vi "Load Layout.vi"(7 "SP_Main":refnum<vi>, 8 "error in (no error)":errorcluster, 11 "hse-config":refnum<class "config-base.lvclass">) -> (0 "error out":errorcluster, 3 "Layout out":T1)   [LabVIEW 2022 SP3, in "UI Manager.lvlib"]
doc: "Loads all the layout files and references and populates the subpanels as configured in UI Manager.ini\n\n____\nHAMPEL SOFTWARE ENGINEERING v2.6.0 (2023-12-19 10:54)"
uses:
  UI Manager.lvlib
  Layout References--cluster.ctl
  SubPanels--map.ctl
  SubPnl Map References--cluster.ctl
  Libraries/hse-libraries/Source/hse-configuration/config-base/config-base.lvclass
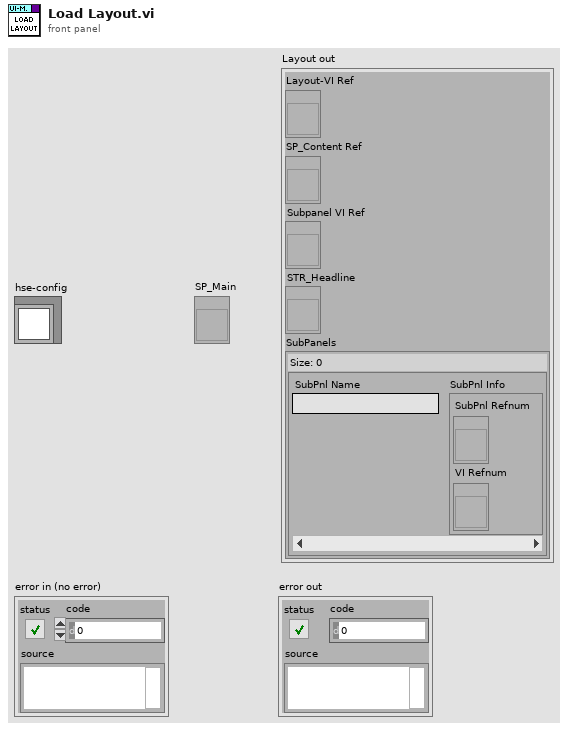
[diagram p1: front panel]
types:
  T1 = typedef "UI Manager.lvlib/Layout References--cluster.ctl" = cluster{"Layout-VI Ref":refnum<vi>, "SP_Content Ref":refnum<vi>, "Subpanel VI Ref":refnum<vi>, "STR_Headline":refnum<vi>, "SubPanels":T2}
  T2 = typedef "UI Manager.lvlib/SubPanels--map.ctl" = map{string, T3}
  T3 = typedef "UI Manager.lvlib/SubPnl Map References--cluster.ctl" = cluster{"SubPnl Refnum":refnum<vi>, "VI Refnum":refnum<vi>}
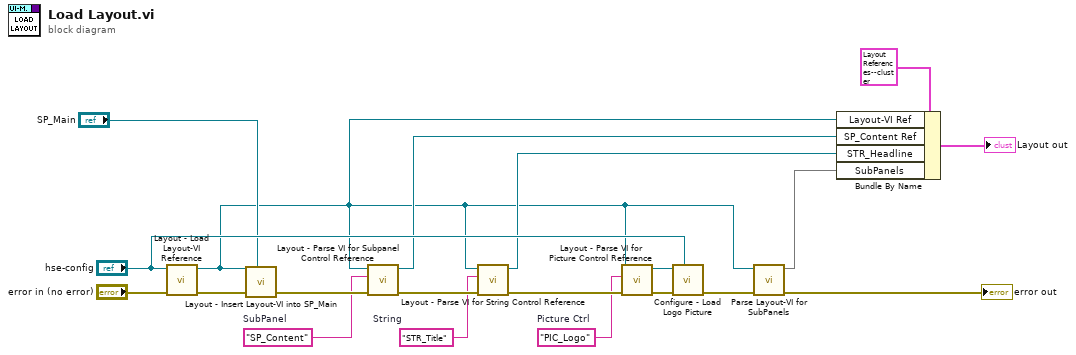
[diagram p0: block diagram]
diagram:
  w6 = "PIC_Logo"  # Picture Ctrl
  w9 = "STR_Title"  # String
  w16 = "SP_Content"  # SubPanel
  n1 = call "Layout - Load Layout-VI Reference.vi"("error in (no error)"="error in (no error)", "hse-config"="hse-config") -> ("error out"=w17:errorcluster, "Layout-VI Ref"=w2:refnum<vi>)  [unwired: 8 in]
  n2 = call "Layout - Insert Layout-VI into SP_Main.vi"("SubPanel in"="SP_Main", "error in (no error)"=w17, "Layout-VI Ref"=w2) -> ("error out"=w18:errorcluster)  [unwired: 8 in]
  n3 = call "Layout - Parse VI for Subpanel Control Reference.vi"("error in (no error)"=w18, "SubPanel Label"=w16, "VI in"=w2) -> ("error out"=w15:errorcluster, "SubPanel Ref"=w19:refnum<vi>)  [unwired: 7 in]
  n4 = call "Layout - Parse VI for String Control Reference.vi"("error in (no error)"=w15, "String Label"=w9, "VI in"=w2) -> ("error out"=w10:errorcluster, "String Reference"=w8:refnum<vi>)  [unwired: 7 in]
  n5 = call "Layout - Parse VI for Picture Control Reference.vi"("error in (no error)"=w10, "Picture Control Label"=w6, "VI in"=w2) -> ("error out"=w7:errorcluster, "Picture Control Ref"=w5:refnum<vi>)  [unwired: 7 in]
  n6 = call "Configure - Load Logo Picture.vi"("hse-config"="hse-config", "error in (no error)"=w7, "Picture Control Ref"=w5) -> ("error out"=w4:errorcluster)  [unwired: 8 in]
  n7 = call "Parse Layout-VI for SubPanels.vi"("error in (no error)"=w4, "Layout-VI Ref"=w2) -> ("error out"=→"error out":errorcluster, "SubPanels"=w1:T2)  [unwired: 8 in]
  n8 = Bundle By Name(cluster=T1 {"Layout-VI Ref"=refnum, "SP_Content Ref"=refnum, "Subpanel VI Ref"=refnum, "STR_Headline"=refnum, "SubPanels"={}} ("Layout out"), "Layout-VI Ref"=w2, "SP_Content Ref"=w19, "STR_Headline"=w8, "SubPanels"=w1) -> (→"Layout out":T1)
